vi "refereeToEnumCommand.vi"(8 "error in (no error)":errorcluster, 9 "touch":bool, 10 "IA State Input":T1, 11 "Referee in":refnum<class "Referee.lvclass">) -> (0 "error out":errorcluster, 3 "Referee out":refnum<class "Referee.lvclass">)   [LabVIEW 2018, in "Referee.lvclass"]
uses:
  Referee.lvclass
  Communication_class/Paths/Convert AI Robot to Robot Command Folder/Core/AI Robot.ctl
  Communication_class/Paths/Convert AI Robot to Robot Command Folder/Intel/Functions Enum.ctl
  Communication_class/Paths/Convert AI Robot to Robot Command Folder/Intel/AttackerStates.ctl
  Communication_class/Paths/Convert AI Robot to Robot Command Folder/Path Planning/RRT/PathDests.ctl
  Communication_class/Paths/Convert AI Robot to Robot Command Folder/Path Planning/RRT/PathDest.ctl
  Communication_class/Paths/MessageAI_State Folder/Core/Field Size.ctl
  command_interpreted.ctl
  Referee.lvclass/Referee.ctl
  Write command_interpreted.vi
  Write command_from_referee.vi
  Write enemy_goalie_id.vi
  Write our_goalie_id.vi
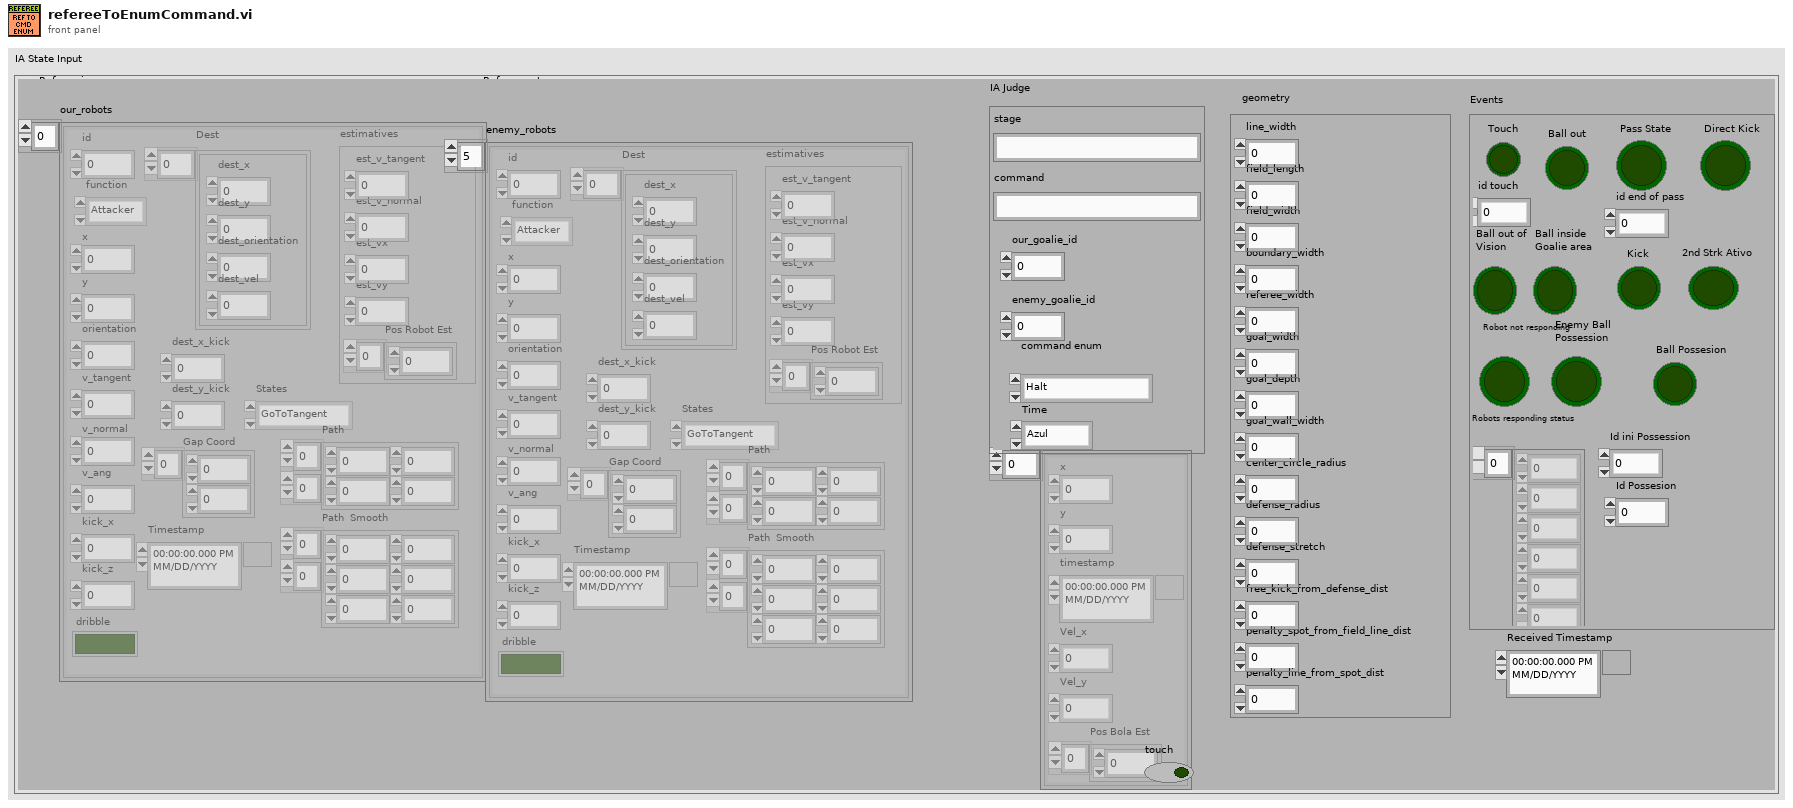
[diagram p1: front panel]
types:
  T1 = typedef "AI Input.ctl" = cluster{"our_robots":T2[], "enemy_robots":T2[], "balls":T7[], "geometry":T8, "IA Judge":T9, "Received Timestamp":timestamp, "Events":T11}
  T2 = typedef "AI Robot.ctl" = cluster{"id":u32, "function":T3, "x":dbl, "y":dbl, "orientation":dbl, "v_tangent":dbl, "v_normal":dbl, "v_ang":dbl, "kick_x":dbl, "kick_z":dbl, "dribble":bool, "Timestamp":timestamp, "estimatives":cluster{"est_v_tangent":dbl, "est_v_normal":dbl, "est_vx":dbl, "est_vy":dbl, "Pos Robot Est":dbl[]}, "dest_x_kick":dbl, "dest_y_kick":dbl, "Gap Coord":dbl[], "States":T4, "Path ":dbl[][], "Path  Smooth":dbl[][], "Dest":T5}
  T3 = typedef "Functions Enum.ctl" = enum16{"2nd Striker", "Attacker", "Goalie", "Defender", "Striker", "Goto 0", "Dummy", "Kicker", "ZigZag 0", "ZigZag 1", "ZigZag 2", "ZigZag 3", "ZigZag 4", "ZigZag 5", "ZigZag 6", "ZigZag 7", "ZigZag 8", ""}
  T4 = typedef "AttackerStates.ctl" = enum16{"Pass", "GoToTangent", "BallGetting", "GoToKick", ""}
  T5 = typedef "PathDests.ctl" = T6[]
  T6 = typedef "PathDest.ctl" = cluster{"dest_x":dbl, "dest_y":dbl, "dest_orientation":dbl, "dest_vel":dbl}
  T7 = typedef "AI Ball.ctl" = cluster{"x":dbl, "y":dbl, "timestamp":timestamp, "Vel_x":dbl, "Vel_y":dbl, "Pos Bola Est":dbl[]}
  T8 = typedef "Field Size.ctl" = cluster{"line_width":u32, "field_length":u32, "field_width":u32, "boundary_width":u32, "referee_width":u32, "goal_width":u32, "goal_depth":u32, "goal_wall_width":u32, "center_circle_radius":u32, "defense_radius":u32, "defense_stretch":u32, "free_kick_from_defense_dist":u32, "penalty_spot_from_field_line_dist":u32, "penalty_line_from_spot_dist":u32}
  T9 = typedef "AI Judge.ctl" = cluster{"stage":string, "command":string, "our_goalie_id":dbl, "enemy_goalie_id":dbl, "command enum":T10, "Time":enum16{"Azul", "Amarelo"}}
  T10 = typedef "Command Enum.ctl" = enum16{"Halt", "Stop", "Force Start", "PKA Normal Start", "Prepare Kickoff Ally", "PKE Normal Start", "Prepare Kickoff Enemy", "Prepare Penalty Ally", "PPA Normal Start", "Prepare Penalty Enemy", "PPE Normal Start", "Direct Free Enemy", "Direct Free Ally", "Indirect Free Enemy", "Indirect Free Ally", "Timeout Enemy", "Timeout Ally", "Goal Enemy", "Goal Ally", "Ball Placement Enemy", "Ball Placement Ally", "Normal Half Time", "Extra Time Break", "Extra Half Time", "None", "Post Game"}
  T11 = typedef "Events.ctl" = cluster{"Touch":bool, "Ball out":bool, "id touch":dbl, "Ball out of \nVision":bool, "Ball inside \nGoalie area":bool, "Robot not responding":bool, "Robots responding status":dbl[], "Enemy Ball \nPossession":bool, "Pass State":bool, "id end of pass":dbl, "Kick":bool, "Id ini Possession":dbl, "Ball Possesion":bool, "Id Possesion":dbl, "Direct Kick":bool, "2nd Strk Ativo":bool}
  T12 = typedef "command_interpreted.ctl" = enum16{"Goal Ally", "Goal Enemy", "Ball Placement Enemy", "Ball Placement Ally", "Normal Half Time", "Extra Time  Break", "Extra Half Time", "None", "Post Game", "PKA Normal Start", "Prepare Kickoff Ally", "PKE Normal Start", "Prepare Kickoff Enemy", "Force Start", "Halt", "Timeout", "Prepare Penalty Ally", "Prepare Penalty Enemy", "PPA NormalStart", "PPE Normal Start", "Indirect Free Ally", "Direct Free Enemy", "Direct Free Ally", "Indirect Free Enemy", "Stop"}
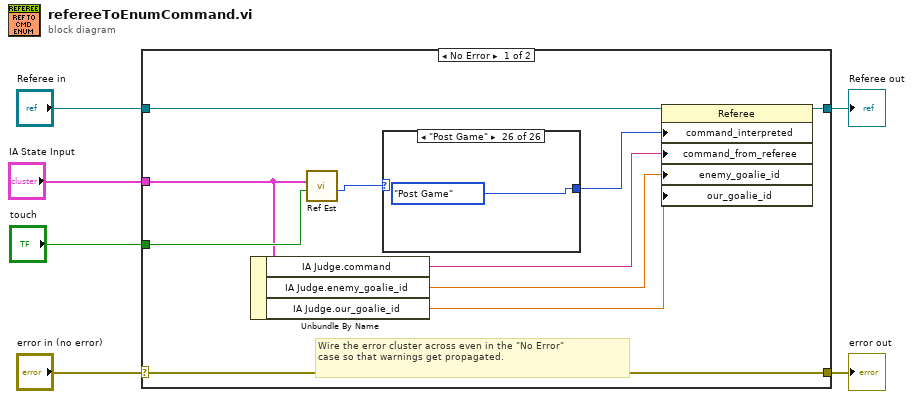
[diagram p0: block diagram]
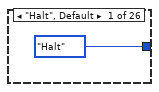
[diagram p2: hidden frame]
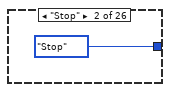
[diagram p3: hidden frame]
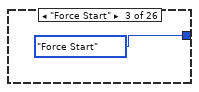
[diagram p4: hidden frame]
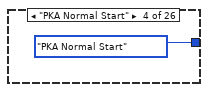
[diagram p5: hidden frame]
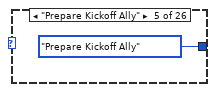
[diagram p6: hidden frame]
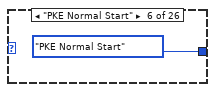
[diagram p7: hidden frame]
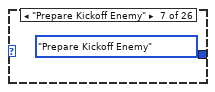
[diagram p8: hidden frame]
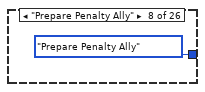
[diagram p9: hidden frame]
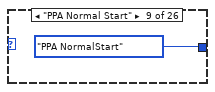
[diagram p10: hidden frame]
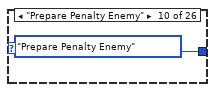
[diagram p11: hidden frame]
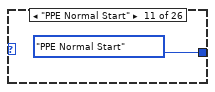
[diagram p12: hidden frame]
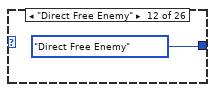
[diagram p13: hidden frame]
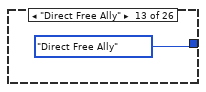
[diagram p14: hidden frame]
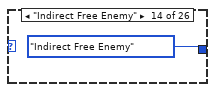
[diagram p15: hidden frame]
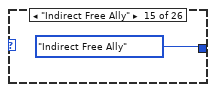
[diagram p16: hidden frame]
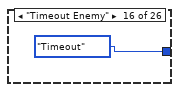
[diagram p17: hidden frame]
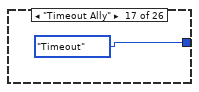
[diagram p18: hidden frame]
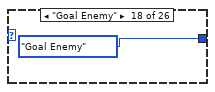
[diagram p19: hidden frame]
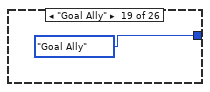
[diagram p20: hidden frame]
diagram:
  n1 = case shown="No Error" "error in (no error)" {
    selector: "error in (no error)" -> [w16 w44]
    tunnel: [w16 w44] -> w5
    tunnel: [w15 w43] -> w3
    tunnel: "Referee in" -> [w14 w43]
    tunnel: "IA State Input" -> [w10 _]
    tunnel: "touch" -> [w13 _]
    frame No Error {
      # "Wire the error cluster across even in the \"No Error\"\ncase so that warnings get propagated."
      n2 = Unbundle By Name(w10) -> ("IA Judge.command"=w9:string, "IA Judge.enemy_goalie_id"=w8:dbl, "IA Judge.our_goalie_id"=w7:dbl)
      n3 = call "Ref Est.vi"("touch"=w13, "IA State Input"=w10) -> ("IA command"=w12:T10)  [unwired: 8 in, 1 out]
      n4 = case shown="\"Post Game\"" w12 {
        tunnel: [command_interpreted."Halt" ("command_interpreted") command_interpreted."Stop" ("command_interpreted") command_interpreted."Force Start" ("command_interpreted") command_interpreted."PKA Normal Start" ("command_interpreted") command_interpreted."Prepare Kickoff Ally" ("command_interpreted") command_interpreted."PKE Normal Start" ("command_interpreted") command_interpreted."Prepare Kickoff Enemy" ("command_interpreted") command_interpreted."Prepare Penalty Ally" ("command_interpreted") command_interpreted."PPA NormalStart" ("command_interpreted") command_interpreted."Prepare Penalty Enemy" ("command_interpreted") command_interpreted."PPE Normal Start" ("command_interpreted") command_interpreted."Direct Free Enemy" ("command_interpreted") command_interpreted."Direct Free Ally" ("command_interpreted") command_interpreted."Indirect Free Enemy" ("command_interpreted") command_interpreted."Indirect Free Ally" ("command_interpreted") command_interpreted."Timeout" ("command_interpreted") command_interpreted."Timeout" ("command_interpreted") command_interpreted."Goal Enemy" ("command_interpreted") command_interpreted."Goal Ally" ("command_interpreted") command_interpreted."Ball Placement Enemy" ("command_interpreted") command_interpreted."Ball Placement Ally" ("command_interpreted") command_interpreted."Normal Half Time" ("command_interpreted") command_interpreted."Extra Time  Break" ("command_interpreted") command_interpreted."Extra Half Time" ("command_interpreted") command_interpreted."None" ("command_interpreted") command_interpreted."Post Game" ("command_interpreted")] -> w11
        frame "Halt", Default {
        }
        frame "Stop" {
        }
        frame "Force Start" {
        }
        frame "PKA Normal Start" {
        }
        frame "Prepare Kickoff Ally" {
        }
        frame "PKE Normal Start" {
        }
        frame "Prepare Kickoff Enemy" {
        }
        frame "Prepare Penalty Ally" {
        }
        frame "PPA Normal Start" {
        }
        frame "Prepare Penalty Enemy" {
        }
        frame "PPE Normal Start" {
        }
        frame "Direct Free Enemy" {
        }
        frame "Direct Free Ally" {
        }
        frame "Indirect Free Enemy" {
        }
        frame "Indirect Free Ally" {
        }
        frame "Timeout Enemy" {
        }
        frame "Timeout Ally" {
        }
        frame "Goal Enemy" {
        }
        frame "Goal Ally" {
        }
        frame "Ball Placement Enemy" {
        }
        frame "Ball Placement Ally" {
        }
        frame "Normal Half Time" {
        }
        frame "Extra Time Break" {
        }
        frame "Extra Half Time" {
        }
        frame "None" {
        }
        frame "Post Game" {
        }
      }
      n5 = property class="Referee"(reference=w14, "command_interpreted"=w11, "command_from_referee"=w9, "enemy_goalie_id"=w8, "our_goalie_id"=w7) -> (reference out=w15:refnum<class "Referee.lvclass">)  [unwired: 1 in, 1 out]
    }
    frame Error {
    }
  }
  "error out" <- w5
  "Referee out" <- w3
